vi "CANopenReadEncoder.vi"() -> ()   [LabVIEW 2020]
uses:
  <vilib>/Platform/TimedLoop/XDataNode/timing_clust.ctl
  <vilib>/Platform/TimedLoop/XDataNode/nitl_modes.ctl
  <vilib>/Platform/TimedLoop/XDataNode/wakeup.ctl
  <vilib>/CANopenLib/CANOPEN.llb/CANopen Interface Create.vi
  <vilib>/CANopenLib/CANOPEN.llb/CANopen TPDO Create.vi
  <vilib>/CANopenLib/CANOPEN.llb/CANopen TPDO Start.vi
  <vilib>/CANopenLib/CANOPEN.llb/CANopen Fetch from Data [U32].vi
  <vilib>/CANopenLib/CANOPEN.llb/CANopen TPDO Close.vi
  <vilib>/CANopenLib/CANOPEN.llb/CANopen Interface Close.vi
  <vilib>/Platform/TimedLoop/XDataNode/XDataNode.xnode
  <vilib>/Platform/TimedLoop/XDataNode/XDNodeRunTimeDep.lvlib
panel:
  in  "buffer size (0) 3":u16=10
  in  "period (ms) 3":i64=1
  in  "stop 3":bool
  out "New data? 3":bool
  out "timestamp 3":timestamp
  out "当前位置 3":u32
  out "基座原始角度值":dbl
  out "TPDO Data 3":u8[](array[numeric])
  out "基座角度值":dbl
  in  "PDO channel 3":u8(ring) items=["PDO 1", "PDO 2", "PDO 3", "PDO 4"]
  in  "node-ID 3":u8=3 min=1 max=127 step=1
  in  "buffer size (0) 2":u16=10
  in  "period (ms) 2":i64=1
  in  "stop 2":bool
  out "New data? 2":bool
  out "timestamp 2":timestamp
  out "当前位置 2":u32
  out "大臂原始角度值":dbl
  out "TPDO Data 2":u8[](array[numeric])
  out "大臂角度值":dbl
  in  "PDO channel 2":u8(ring) items=["PDO 1", "PDO 2", "PDO 3", "PDO 4"]
  in  "node-ID 2":u8=2 min=1 max=127 step=1
  out "三角形角度":dbl
  out "手腕角度值":dbl
  out "TPDO Data":u8[](array[numeric])
  out "手腕原始角度值":dbl
  out "当前位置":u32
  in  "buffer size (0)":u16=10
  in  "period (ms)":i64=1
  in  "stop":bool
  out "New data?":bool
  out "timestamp":timestamp
  in  "PDO channel":u8(ring) items=["PDO 1", "PDO 2", "PDO 3", "PDO 4"]
  in  "node-ID":u8=1 min=1 max=127 step=1
  in  "baud rate":u32(ring)=2 items=["1 Mbit/s"=0, "800 kbit/s"=1, "500 kbit/s"=2, "250 kbit/s"=3, "125 kbit/s"=4, "50 kbit/s"=6, "20 kbit/s"=7, "10 kbit/s"=8]
  in  "CANopen interface":u32(ring)=2 items=["CANopen01", "CANopen02", "CANopen03", "CANopen04", "CANopen05", "CANopen06", "CANopen07", "CANopen08", "CANopen09", "CANopen10", "CANopen11", "CANopen12", "CANopen13", "CANopen14", "CANopen15", "CANopen16", "CANopen17", "CANopen18", "CANopen19", "CANopen20", "CANopen21", "CANopen22", "CANopen23", "CANopen24", "CANopen25", "CANopen26", "CANopen27", "CANopen28", "CANopen29", "CANopen30", "CANopen31", "CANopen32"]
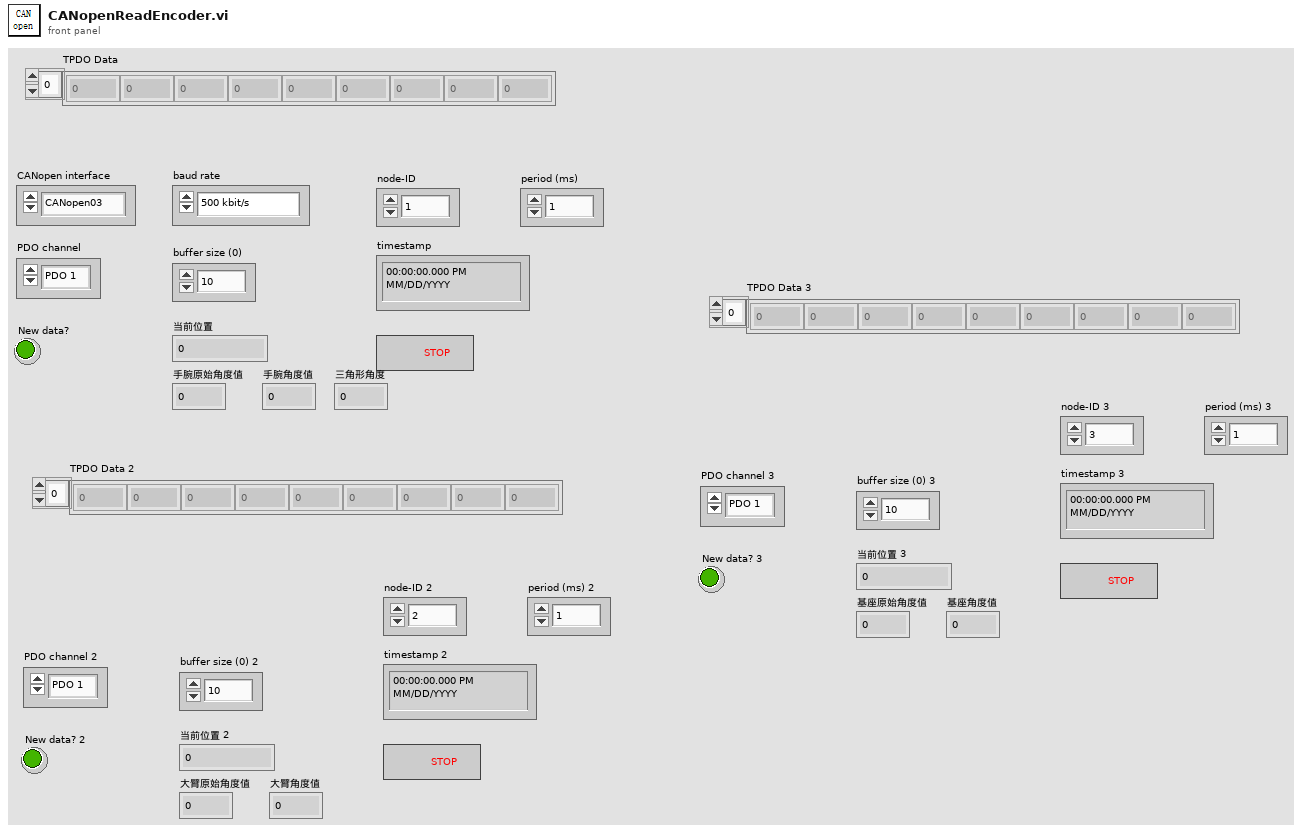
[diagram p1: front panel]
types:
  T1 = typedef "XDNodeRunTimeDep.lvlib/timing_clust.ctl" = cluster{"Expected End [f-1]":u64, "Actual End [f-1]":u64, "Finished Late? [f-1]":bool, "Expected End [i-1]":u64, "Actual End [i-1]":u64, "Finished Late? [i-1]":bool, "Expected Start [i]":u64, "Actual Start [i]":u64, "Expected Start [f]":u64, "Actual Start [f]":u64, "Source Name":string, "Structure Name":string, "Period":i64, "Deadline":i64, "Offset":i64, "Start":i64, "Priority":i32, "Timeout":i32, "Mode":T2, "Wakeup Reason":T3, "Error":errorcluster, "Source Type":string, "Secondary Source Type":string, "Global End Time":u64, "Global Start Time":u64, "Frame Duration":u64, "Iteration Duration":u64, "Assigned CPU":i32, "I/O Scan Engine Mode":u32}
  T2 = typedef "XDNodeRunTimeDep.lvlib/nitl_modes.ctl" = enum32{"No Change", "Process missed periods, maintain original phase", "Discard missed periods, maintain original phase", "Process missed periods, ignore original phase", "Discard missed periods, ignore original phase"}
  T3 = typedef "XDNodeRunTimeDep.lvlib/wakeup.ctl" = enum32{"Normal", "Aborted", "Asynchronous wakeup", "Timing source error", "Timed loop error", "Timeout"}
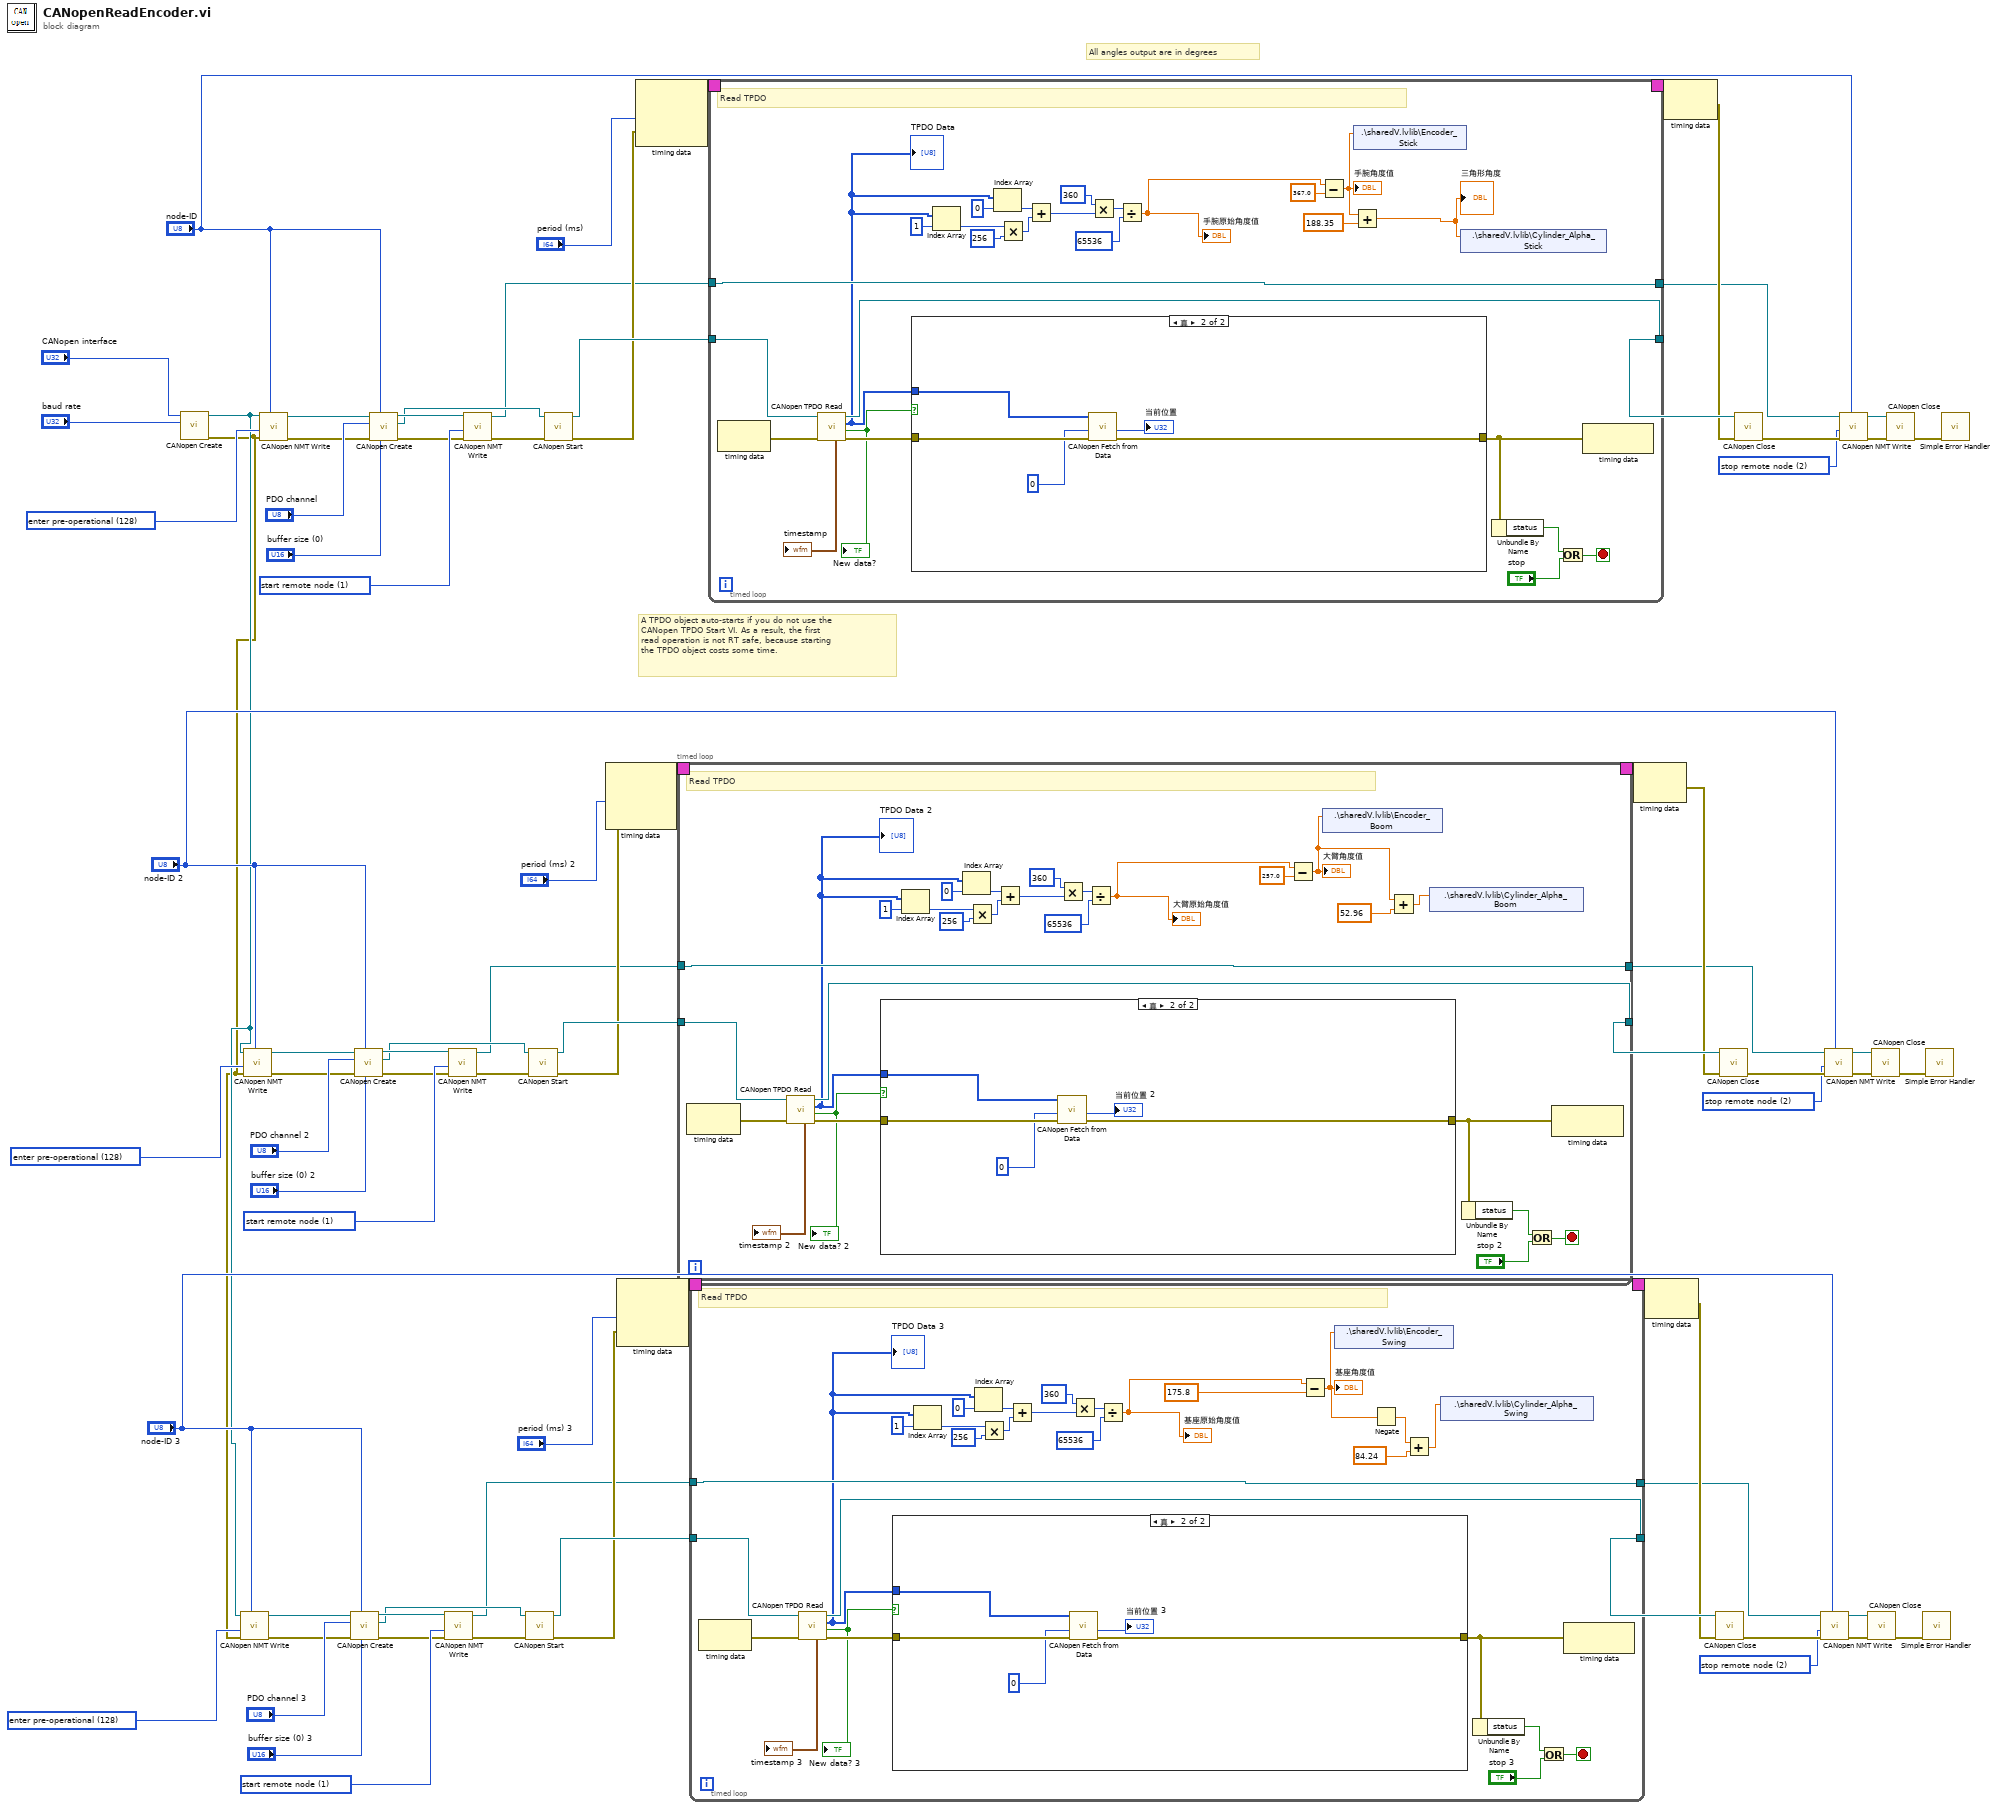
[diagram p0: block diagram]
diagram:
  w15 = u16 1 items=["start remote node"=1, "stop remote node"=2, "enter pre-operational"=128, "reset node"=129, "reset communication"=130] ("command")
  w19 = u16 2 items=["start remote node"=1, "stop remote node"=2, "enter pre-operational"=128, "reset node"=129, "reset communication"=130] ("command")
  w26 = u16 128 items=["start remote node"=1, "stop remote node"=2, "enter pre-operational"=128, "reset node"=129, "reset communication"=130] ("command")
  w40 = u16 1 items=["start remote node"=1, "stop remote node"=2, "enter pre-operational"=128, "reset node"=129, "reset communication"=130] ("command")
  w44 = u16 2 items=["start remote node"=1, "stop remote node"=2, "enter pre-operational"=128, "reset node"=129, "reset communication"=130] ("command")
  w51 = u16 128 items=["start remote node"=1, "stop remote node"=2, "enter pre-operational"=128, "reset node"=129, "reset communication"=130] ("command")
  w65 = u16 1 items=["start remote node"=1, "stop remote node"=2, "enter pre-operational"=128, "reset node"=129, "reset communication"=130] ("command")
  w69 = u16 2 items=["start remote node"=1, "stop remote node"=2, "enter pre-operational"=128, "reset node"=129, "reset communication"=130] ("command")
  w76 = u16 128 items=["start remote node"=1, "stop remote node"=2, "enter pre-operational"=128, "reset node"=129, "reset communication"=130] ("command")
  # "All angles output are in degrees"
  # "A TPDO object auto-starts if you do not use the \nCANopen TPDO Start VI. As a result, the first \nread operation is not RT safe, because starting \nthe TPDO object costs some time."
  n1 = call-poly <vilib>:"CANopen Create.vi"("baud rate"="baud rate", "interface name"="CANopen interface") -> ("error out"=w1:errorcluster, "interface object out"=w2:refnum<k20>)  [unwired: 8 in]
  n2 = call <vilib>:"CANopen NMT Write.vi"("node-ID (0)"="node-ID 3", "error in (no error)"=w1, "command"=w26, "interface object in"=w2) -> ("error out"=w5:errorcluster, "interface object out"=w6:refnum<k20>)  [unwired: 6 in]
  n3 = call <vilib>:"CANopen NMT Write.vi"("node-ID (0)"="node-ID 2", "error in (no error)"=w1, "command"=w51, "interface object in"=w2) -> ("error out"=w30:errorcluster, "interface object out"=w31:refnum<k20>)  [unwired: 6 in]
  n4 = call <vilib>:"CANopen NMT Write.vi"("node-ID (0)"="node-ID", "error in (no error)"=w1, "command"=w76, "interface object in"=w2) -> ("error out"=w55:errorcluster, "interface object out"=w56:refnum<k20>)  [unwired: 6 in]
  n5 = call-poly <vilib>:"CANopen Create.vi"("buffer size (0)"="buffer size (0) 3", "node-ID"="node-ID 3", "error in (no error)"=w5, "PDO channel"="PDO channel 3", "interface object in"=w6) -> ("error out"=w13:errorcluster, "TPDO object out"=w12:refnum<k20>, "interface object out"=w16:refnum<k20>)  [unwired: 4 in]
  n6 = call-poly <vilib>:"CANopen Create.vi"("buffer size (0)"="buffer size (0) 2", "node-ID"="node-ID 2", "error in (no error)"=w30, "PDO channel"="PDO channel 2", "interface object in"=w31) -> ("error out"=w38:errorcluster, "TPDO object out"=w37:refnum<k20>, "interface object out"=w41:refnum<k20>)  [unwired: 4 in]
  n7 = call-poly <vilib>:"CANopen Create.vi"("buffer size (0)"="buffer size (0)", "node-ID"="node-ID", "error in (no error)"=w55, "PDO channel"="PDO channel", "interface object in"=w56) -> ("error out"=w63:errorcluster, "TPDO object out"=w62:refnum<k20>, "interface object out"=w66:refnum<k20>)  [unwired: 4 in]
  n8 = call <vilib>:"CANopen NMT Write.vi"("error in (no error)"=w13, "command"=w15, "interface object in"=w16) -> ("error out"=w14:errorcluster, "interface object out"=w8:refnum<k20>)  [unwired: 7 in]
  n9 = call <vilib>:"CANopen NMT Write.vi"("error in (no error)"=w38, "command"=w40, "interface object in"=w41) -> ("error out"=w39:errorcluster, "interface object out"=w33:refnum<k20>)  [unwired: 7 in]
  n10 = call <vilib>:"CANopen NMT Write.vi"("error in (no error)"=w63, "command"=w65, "interface object in"=w66) -> ("error out"=w64:errorcluster, "interface object out"=w58:refnum<k20>)  [unwired: 7 in]
  n11 = call-poly <vilib>:"CANopen Start.vi"("error in (no error)"=w14, "TPDO object in"=w12) -> ("error out"=w11:errorcluster, "TPDO object out"=w23:refnum<k20>)  [unwired: 8 in]
  n12 = call-poly <vilib>:"CANopen Start.vi"("error in (no error)"=w39, "TPDO object in"=w37) -> ("error out"=w36:errorcluster, "TPDO object out"=w48:refnum<k20>)  [unwired: 8 in]
  n13 = call-poly <vilib>:"CANopen Start.vi"("error in (no error)"=w64, "TPDO object in"=w62) -> ("error out"=w61:errorcluster, "TPDO object out"=w73:refnum<k20>)  [unwired: 8 in]
  n14 = node-c288("period (ms) 2", w36) -> (w53:T1)  [unwired: 1 in]
  n15 = node-c288("period (ms) 3", w11) -> (w28:T1)  [unwired: 1 in]
  n16 = node-c288("period (ms)", w61) -> (w79:T1)  [unwired: 1 in]
  n17 = timed-loop {
    tunnel: [w103] -> w50
    tunnel: w48 -> [w106]
    timing: w53 -> [_]
    timing-out: [_] -> w52
    tunnel: w33 -> [w97]
    tunnel: [w97] -> w32
    stop <- w101 stop-if-true
    # "Read TPDO"
    n18 = node-c288() -> (w99:errorcluster)  [unwired: 1 in]
    n19 = call <vilib>:"CANopen TPDO Read.vi"("error in (no error)"=w99, "TPDO object in"=w106) -> ("error out"=w104:errorcluster, "new data?"=w100:bool, "data"=w91:u8[], "TPDO object out"=w103:refnum<k20>, "timestamp"=→"timestamp 2":timestamp)  [unwired: 5 in]
    "New data? 2" <- w100
    "TPDO Data 2" <- w91
    n20 = case shown="真" w100 {
      tunnel: w104 -> [w112 w117]
      tunnel: w91 -> [_ w116]
      tunnel: [w112 w115] -> w96
      frame False {
      }
      frame True {
        n21 = call-poly <vilib>:"CANopen Fetch from Data.vi"("error in (no error)"=w117, "offset (0)"=u32 0, "CANopen data in"=w116) -> ("error out"=w115:errorcluster, "unsigned 32-bit integer"=→"当前位置 2":u32)  [unwired: 6 in, 1 out]
      }
    }
    n22 = Index Array(array=w91, index=1) -> (element=w88:u8)
    n23 = Index Array(array=w91, index=0) -> (element=w87:u8)
    n24 = Multiply(x=w88, y=256) -> (x*y=w86:i32)
    n25 = Add(x=w87, y=w86) -> (x+y=w85:i32)
    n26 = Multiply(x=u32 360, y=w85) -> (x*y=w94:u32)
    n27 = Divide(x=w94, y=u32 65536) -> (x/y=w83:dbl)
    "大臂原始角度值" <- w83
    n28 = Subtract(x=w83, y=257.0) -> (x-y=w81:dbl)
    "大臂角度值" <- w81
    n29 = shared-variable ".\\sharedV.lvlib\\Encoder_Boom"(w81) -> ()  [unwired: 1 in, 1 out]
    n30 = Add(x=w81, y=52.96) -> (x+y=w80:dbl)
    n31 = shared-variable ".\\sharedV.lvlib\\Cylinder_Alpha_Boom"(w80) -> ()  [unwired: 1 in, 1 out]
    n32 = Unbundle By Name(w96) -> ("status"=w98:bool)
    n33 = Or(x=w98, y="stop 2") -> (x .or. y?=w101:bool)
    n34 = node-c288(w96) -> ()  [unwired: 1 out]
  }
  n35 = timed-loop {
    tunnel: [w142] -> w25
    tunnel: w23 -> [w145]
    timing: w28 -> [_]
    timing-out: [_] -> w27
    tunnel: w8 -> [w136]
    tunnel: [w136] -> w7
    stop <- w140 stop-if-true
    # "Read TPDO"
    n36 = node-c288() -> (w138:errorcluster)  [unwired: 1 in]
    n37 = call <vilib>:"CANopen TPDO Read.vi"("error in (no error)"=w138, "TPDO object in"=w145) -> ("error out"=w143:errorcluster, "new data?"=w139:bool, "data"=w130:u8[], "TPDO object out"=w142:refnum<k20>, "timestamp"=→"timestamp 3":timestamp)  [unwired: 5 in]
    "New data? 3" <- w139
    "TPDO Data 3" <- w130
    n38 = case shown="真" w139 {
      tunnel: w143 -> [w151 w156]
      tunnel: w130 -> [_ w155]
      tunnel: [w151 w154] -> w135
      frame False {
      }
      frame True {
        n39 = call-poly <vilib>:"CANopen Fetch from Data.vi"("error in (no error)"=w156, "offset (0)"=u32 0, "CANopen data in"=w155) -> ("error out"=w154:errorcluster, "unsigned 32-bit integer"=→"当前位置 3":u32)  [unwired: 6 in, 1 out]
      }
    }
    n40 = Index Array(array=w130, index=1) -> (element=w127:u8)
    n41 = Index Array(array=w130, index=0) -> (element=w126:u8)
    n42 = Multiply(x=w127, y=256) -> (x*y=w125:i32)
    n43 = Add(x=w126, y=w125) -> (x+y=w124:i32)
    n44 = Multiply(x=u32 360, y=w124) -> (x*y=w133:u32)
    n45 = Divide(x=w133, y=u32 65536) -> (x/y=w122:dbl)
    "基座原始角度值" <- w122
    n46 = Subtract(x=w122, y=175.8) -> (x-y=w119:dbl)
    "基座角度值" <- w119
    n47 = shared-variable ".\\sharedV.lvlib\\Encoder_Swing"(w119) -> ()  [unwired: 1 in, 1 out]
    n48 = Negate(x=w119) -> (-x=w118:dbl)
    n49 = Add(x=w118, y=84.24) -> (x+y=w120:dbl)
    n50 = shared-variable ".\\sharedV.lvlib\\Cylinder_Alpha_Swing"(w120) -> ()  [unwired: 1 in, 1 out]
    n51 = Unbundle By Name(w135) -> ("status"=w137:bool)
    n52 = Or(x=w137, y="stop 3") -> (x .or. y?=w140:bool)
    n53 = node-c288(w135) -> ()  [unwired: 1 out]
  }
  n54 = timed-loop {
    tunnel: [w180] -> w75
    tunnel: w73 -> [w183]
    timing: w79 -> [_]
    timing-out: [_] -> w78
    tunnel: w58 -> [w174]
    tunnel: [w174] -> w57
    stop <- w178 stop-if-true
    # "Read TPDO"
    n55 = node-c288() -> (w176:errorcluster)  [unwired: 1 in]
    n56 = call <vilib>:"CANopen TPDO Read.vi"("error in (no error)"=w176, "TPDO object in"=w183) -> ("error out"=w181:errorcluster, "new data?"=w177:bool, "data"=w168:u8[], "TPDO object out"=w180:refnum<k20>, "timestamp"=→"timestamp":timestamp)  [unwired: 5 in]
    "New data?" <- w177
    "TPDO Data" <- w168
    n57 = case shown="真" w177 {
      tunnel: w181 -> [w189 w194]
      tunnel: w168 -> [_ w193]
      tunnel: [w189 w192] -> w173
      frame False {
      }
      frame True {
        n58 = call-poly <vilib>:"CANopen Fetch from Data.vi"("error in (no error)"=w194, "offset (0)"=u32 0, "CANopen data in"=w193) -> ("error out"=w192:errorcluster, "unsigned 32-bit integer"=→"当前位置":u32)  [unwired: 6 in, 1 out]
      }
    }
    n59 = Index Array(array=w168, index=1) -> (element=w165:u8)
    n60 = Index Array(array=w168, index=0) -> (element=w164:u8)
    n61 = Multiply(x=w165, y=256) -> (x*y=w163:i32)
    n62 = Add(x=w164, y=w163) -> (x+y=w162:i32)
    n63 = Multiply(x=u32 360, y=w162) -> (x*y=w171:u32)
    n64 = Divide(x=w171, y=u32 65536) -> (x/y=w160:dbl)
    "手腕原始角度值" <- w160
    n65 = Subtract(x=w160, y=367.0) -> (x-y=w158:dbl)
    "手腕角度值" <- w158
    n66 = shared-variable ".\\sharedV.lvlib\\Encoder_Stick"(w158) -> ()  [unwired: 1 in, 1 out]
    n67 = Add(x=w158, y=188.35) -> (x+y=w157:dbl)
    "三角形角度" <- w157
    n68 = shared-variable ".\\sharedV.lvlib\\Cylinder_Alpha_Stick"(w157) -> ()  [unwired: 1 in, 1 out]
    n69 = Unbundle By Name(w173) -> ("status"=w175:bool)
    n70 = Or(x=w175, y="stop") -> (x .or. y?=w178:bool)
    n71 = node-c288(w173) -> ()  [unwired: 1 out]
  }
  n72 = node-c288(w52) -> (w35:errorcluster)
  n73 = node-c288(w27) -> (w10:errorcluster)
  n74 = node-c288(w78) -> (w60:errorcluster)
  n75 = call-poly <vilib>:"CANopen Close.vi"("error in (no error)"=w10, "TPDO object in"=w25) -> ("error out"=w20:errorcluster)  [unwired: 9 in]
  n76 = call-poly <vilib>:"CANopen Close.vi"("error in (no error)"=w35, "TPDO object in"=w50) -> ("error out"=w45:errorcluster)  [unwired: 9 in]
  n77 = call-poly <vilib>:"CANopen Close.vi"("error in (no error)"=w60, "TPDO object in"=w75) -> ("error out"=w70:errorcluster)  [unwired: 9 in]
  n78 = call <vilib>:"CANopen NMT Write.vi"("node-ID (0)"="node-ID 3", "error in (no error)"=w20, "command"=w19, "interface object in"=w7) -> ("error out"=w22:errorcluster, "interface object out"=w21:refnum<k20>)  [unwired: 6 in]
  n79 = call <vilib>:"CANopen NMT Write.vi"("node-ID (0)"="node-ID 2", "error in (no error)"=w45, "command"=w44, "interface object in"=w32) -> ("error out"=w47:errorcluster, "interface object out"=w46:refnum<k20>)  [unwired: 6 in]
  n80 = call <vilib>:"CANopen NMT Write.vi"("node-ID (0)"="node-ID", "error in (no error)"=w70, "command"=w69, "interface object in"=w57) -> ("error out"=w72:errorcluster, "interface object out"=w71:refnum<k20>)  [unwired: 6 in]
  n81 = call-poly <vilib>:"CANopen Close.vi"("error in (no error)"=w22, "interface object in"=w21) -> ("error out"=w9:errorcluster)  [unwired: 9 in]
  n82 = call-poly <vilib>:"CANopen Close.vi"("error in (no error)"=w47, "interface object in"=w46) -> ("error out"=w34:errorcluster)  [unwired: 9 in]
  n83 = call-poly <vilib>:"CANopen Close.vi"("error in (no error)"=w72, "interface object in"=w71) -> ("error out"=w59:errorcluster)  [unwired: 9 in]
  n84 = call <vilib>:"Simple Error Handler.vi"("error in (no error)"=w9) -> ()  [unwired: 4 in, 5 out]
  n85 = call <vilib>:"Simple Error Handler.vi"("error in (no error)"=w34) -> ()  [unwired: 4 in, 5 out]
  n86 = call <vilib>:"Simple Error Handler.vi"("error in (no error)"=w59) -> ()  [unwired: 4 in, 5 out]
